vi "PKG_IMC_GetGout.vi"(10 "gout":u16[](array[numeric])=[0, 0, 0, 0, 0, 0, 0, 0, 0, 0, 0, 0, 0, 0, 0, 0, 0, 0, 0, 0, 0, 0, 0, 0, 0, 0, 0, 0, 0, 0, 0, 0, 0, 0, 0, 0, 0, 0, 0, 0, 0, 0, 0, 0, 0, 0, 0, 0], 11 "Handle":u32) -> (1 "function return":i32, 2 "gout out":u16[](array[numeric]), 3 "Handle out":u32)   [LabVIEW 2011, in "IMC_Pkg4xxx.lvlib"]
doc: "PKG_IMC_GetGout(IMC_HANDLE Handle, unsigned short gout[48]);"
uses:
  IMC_Pkg4xxx.lvlib
  IMC_Pkg4xxx.dll
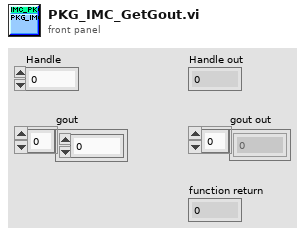
[diagram p1: front panel]
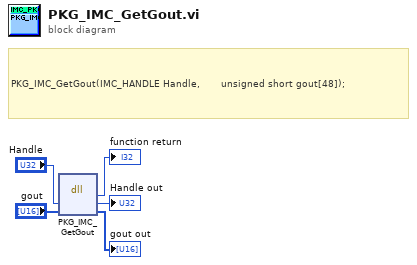
[diagram p0: block diagram]
diagram:
  # "PKG_IMC_GetGout(IMC_HANDLE Handle, \t\t\t\t\t\tunsigned short gout[48]);"
  n1 = dll-call lib="PTH1mabs F光盘刻录\niMC MotionIMCNet_V4.0IMCAppincLabviewIMC_PKG4xxxIMC_PKG4xxx\nIMC_Pkg4xxx.*" fn="PKG_IMC_GetGout"("Handle"="Handle", "gout"="gout") -> (→"function return":i32, "Handle"=→"Handle out":u32, "gout"=→"gout out":u16[])  [unwired: 3 in, 2 out]
